vi "Main_12A_X1.vi"() -> ()   [LabVIEW 2024]
uses:
  Utility/Universal Utility/TypeDefs_Utility/Cluster_Row-Column.ctl
  <vilib>/Utility/miscctls.llb/LVMapReplaceAction.ctl
  Utility/Universal Utility/TypeDefs_Utility/ENUM_4 Directions U-D-L-R.ctl
  01caa875-3ad4-4b16-8180-2387dde84b10.vi
  43e758e7-457a-4b0b-abaa-443db623fd74.vi
panel:
  out "Map 2":map{string, map{T1, u32}[]}(c390)
  out "Perimeter 2":map{T1, u32}[](array[numeric])
  out "Area":i32[](array[numeric])
  out "Plant Array":string[](array[string])
  out "Perimeter":u32[](array[numeric])
  out "Map":map{string, T1[]}(c390)
  in  "Example 3":string="RRRRIICCFF\nRRRRIICCCF\nVVRRRCCFFF\nVVRCCCJFFF\nVVVVCJJCFE\nVVIVCCJJEE\nVVIIICJJEE\nMIIIIIJJEE\nMIIISIJEEE\nMMMISSJEEE"
  in  "Example 2":string="OOOOO\nOXOXO\nOOOOO\nOXOXO\nOOOOO"
  in  "Use Puzzle":bool
  out "Answer":u32
  in  "Puzzle":string="WWWWWWWWWWWWWWWWWWHHHHHHHHHHHBYYYYYYYYYYYJJJJJJJJJJJJJJZLLLLLLLLLLLLLLLLLLLLLLBBYBBBBBBBBTTTTKKKKKKKKKKKKKOOOUUUUUUUUUUUSSSSSSSSSSSSSSSSSSSO\nWWWWWWWWWWWWWWWWWWHEHEHHHHHHBBBYYYYYYYYYYJJJJJJJWJJZJZZZZLLLLLLLLLLLLLLLLLLLLLBBBBBBBBBBBBTTTKKKKKKKKKKKKKOOOUUUUUUUUUUUUSSSSSSSSSSSSSSSSSHH\nWWWWWWWWWWWWWWWWWWWEEEHHHHHBBBBBYYYYYYYYYJYJJJJWWJJZZZZZZLLLFFFLLLFLLLHHHHHHHLBBBBBBBBBBBBTTTKKKKKKKKKKKKKOOOOUUUUUUUUUSSSSSSSSSSSSSSSSSSSHH\nWWWWWWWWWWWWWWWWWEEEEEEEEHHBBBSSYYYYYYYYYYYWWWWWWJJZZZZZZLFLFFFFFLFFFLHHHNHHHHABBBBBBBBBBBTTKKKKKKKKKKKKKKOOOUUUUUUUUUUSSSSSSSSSSSSSSSSSHHHH\nWWWWWWWWWWWWWWGEEEEEEEEHEHHHHHHSYYYY..."
  in  "Example 1":string="AAAA\nBBCD\nBBCC\nEEEC"
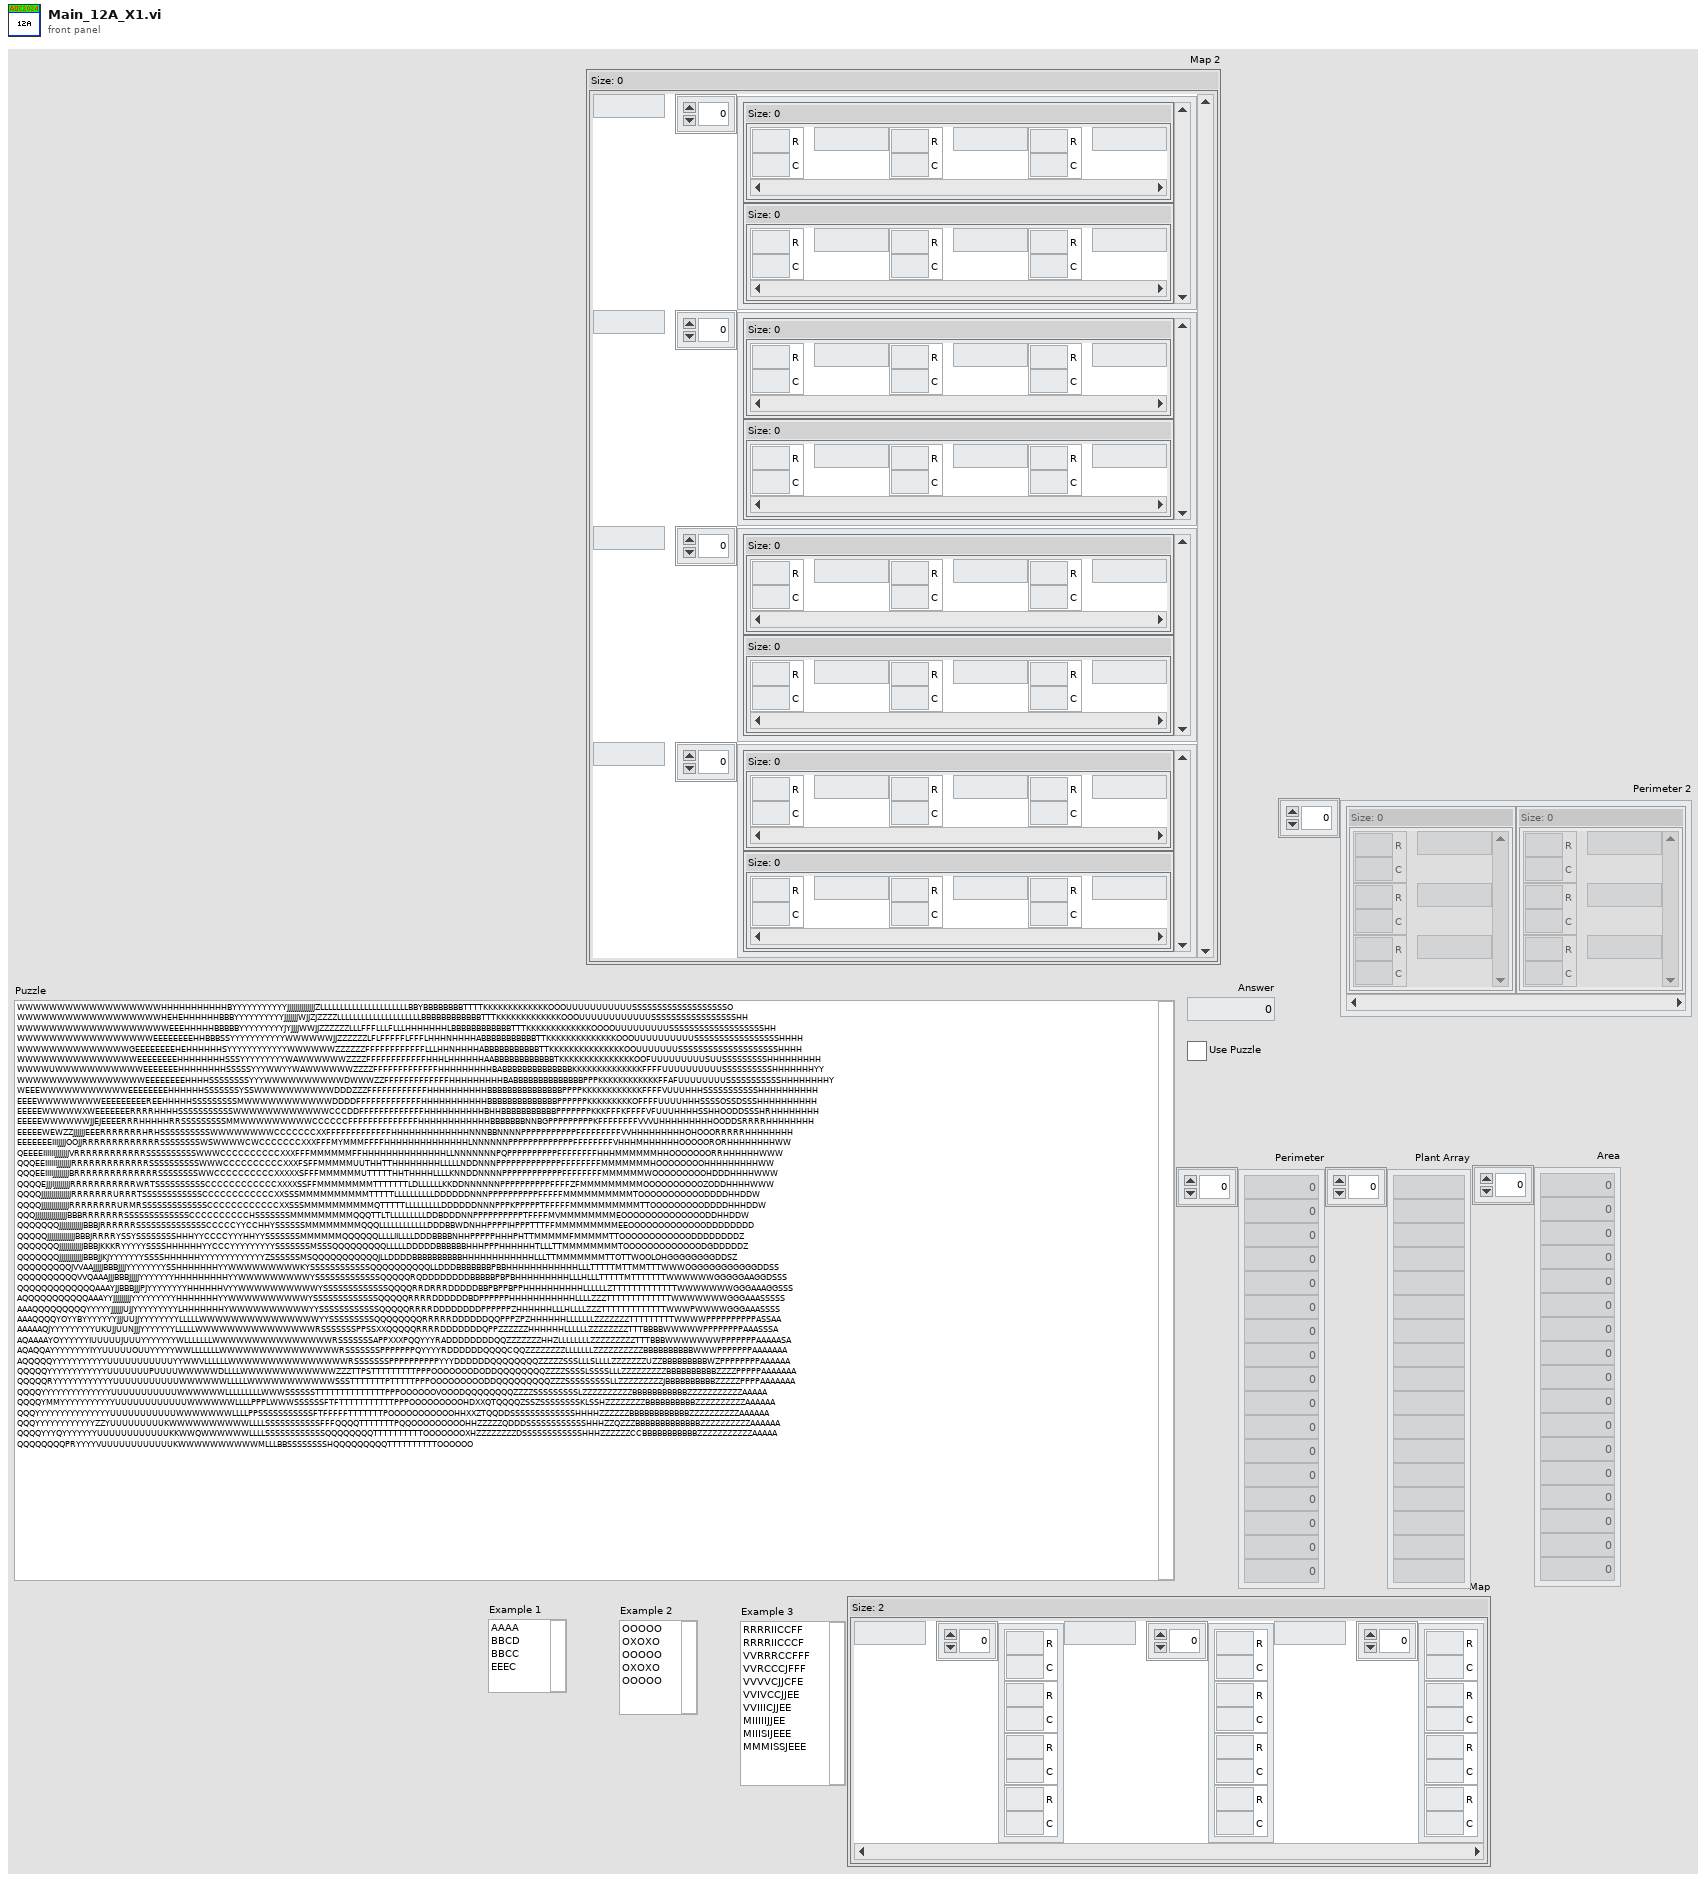
[diagram p1: front panel]
types:
  T1 = typedef "Cluster_Row-Column.ctl" = cluster{"R":i32, "C":i32}
  T2 = typedef "LVMapReplaceAction.ctl" = enum32{"Modify Entry only if found", "Add or Modify Entry", "Delete Entry"}
  T3 = typedef "ENUM_4 Directions U-D-L-R.ctl" = enum16{"Up;-1,0", "Right;0,1", "Down;1,0", "Left;0,-1"}
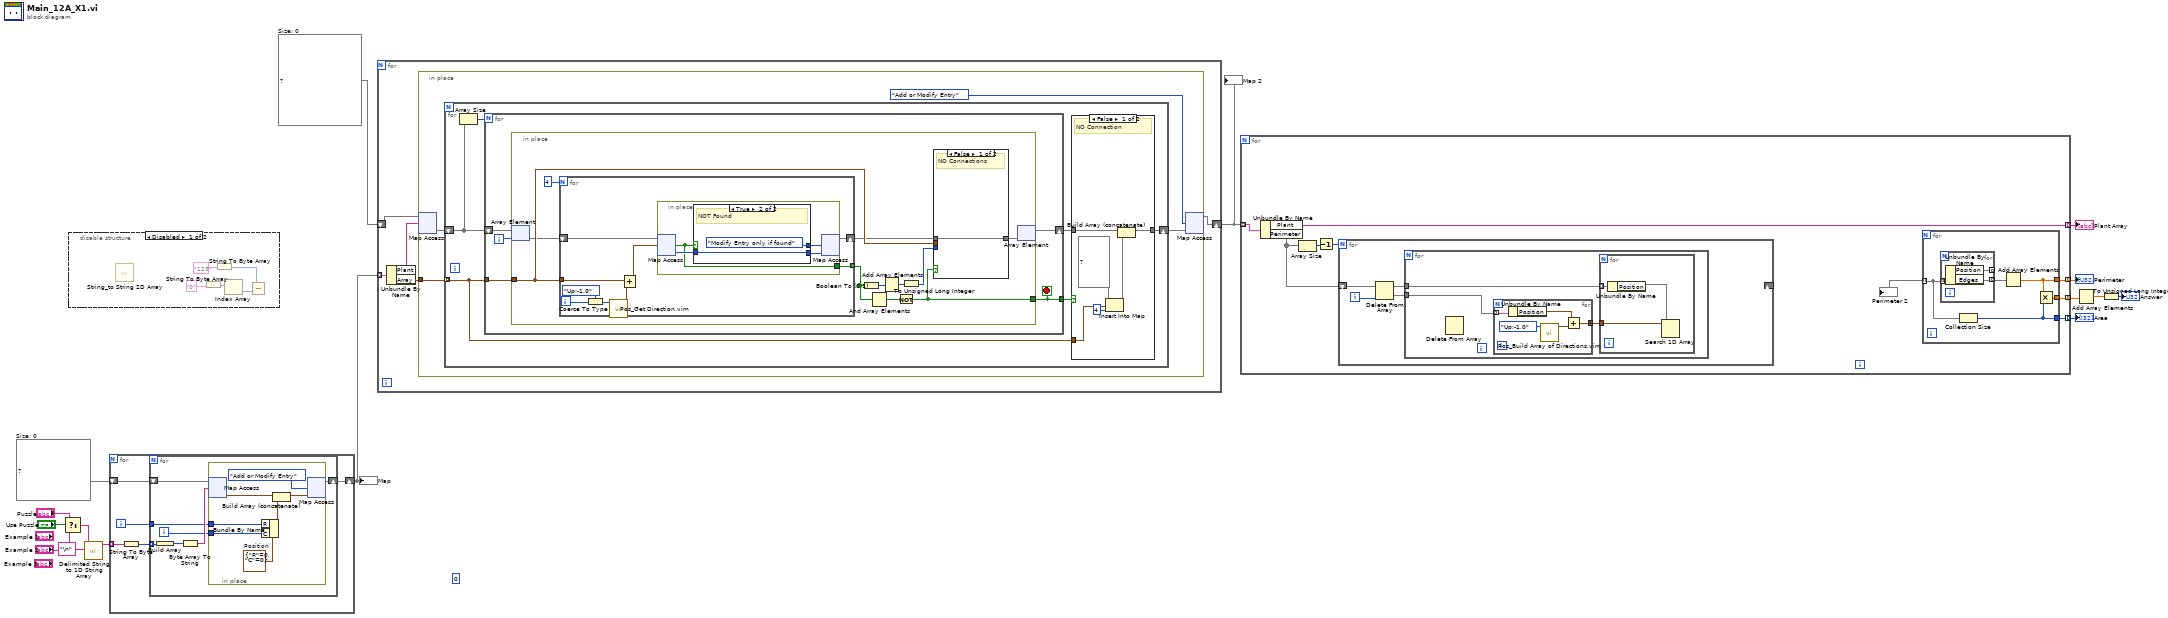
[diagram p0: block diagram]
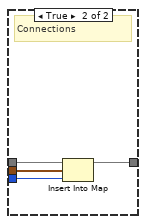
[diagram p3: hidden frame]
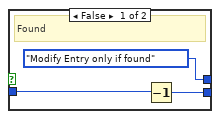
[diagram p4: hidden frame]
diagram:
  w8 = map{string, map{T1, u32}[]} {}  # Size: 0
  w10 = map{string, T1[]} {}  # Size: 0
  (unwired) u32 0 ("number")
  n1 = Select(t="Puzzle", s="Use Puzzle", f="Example 2") -> (s? t:f=w13:string)
  n2 = disable-structure shown="Disabled" {
    frame Disabled {
      n3 = call "String_to String 2D Array.vi"() -> ()  [unwired: 11 in, 1 out]
      n4 = String To Byte Array(string="0") -> (unsigned byte array=w19:u8[])
      n5 = String To Byte Array(string="123") -> (unsigned byte array=w17:u8[])
      n6 = Index Array(array=w19) -> (element=w18:u8)  [unwired: 1 in]
      n7 = Subtract(x=w17, y=w18) -> ()  [unwired: 1 out]
    }
    frame Enabled {
    }
  }
  n8 = call <vilib>:"Delimited String to 1D String Array.vi"("delimiter"="\n" ("delimiter (Tab)"), "delimited string"=w13) -> ("string array"=w15:string[])  [unwired: 9 in]
  n9 = for {
    tunnel: w15 -> [w26] mode=indexing
    shift-right: [w23] -> w9
    shift-left: w10 -> [w24]
    i -> [w22]
    n10 = String To Byte Array(string=w26) -> (unsigned byte array=w25:u8[])
    n11 = for {
      tunnel: w25 -> [w33] mode=indexing
      shift-right: [w30] -> w23
      shift-left: w24 -> [w31]
      tunnel: w22 -> [w28]
      i -> [w27]
      n12 = Build Array(w33) -> (w32:u8[])
      n13 = Byte Array To String(unsigned byte array=w32) -> (string=w29:string)
      n14 = in-place {
        in-place-border: w28 -> [w38]
        in-place-border: w27 -> [w37]
        w39 = T1 {"R"=0, "C"=0}  # Position
        n15 = in-place-map #1(w31, w29) -> (w36:T1[])  [unwired: 1 in, 1 out]
        n16 = Bundle By Name(cluster=w39, "R"=w38, "C"=w37) -> (w34:T1)
        n17 = Build Array (concatenate)(w36, w34) -> (w35:T1[])
        n18 = in-place-map #1(w35, LVMapReplaceAction."Add or Modify Entry" ("action")) -> (w30:map{string, T1[]})  [unwired: 2 out]
      }
    }
  }
  "Map" <- w9
  n19 = for {
    tunnel: w9 -> [w45] mode=indexing
    shift-right: [w43] -> w7
    shift-left: w8 -> [w44]
    n20 = Unbundle By Name(w45) -> ("Plant"=w42:string, "Array"=w41:T1[])
    n21 = in-place {
      in-place-border: w41 -> [w48]
      n22 = in-place-map #2(w44, w42) -> (w47:map{T1, u32}[])  [unwired: 1 in, 1 out]
      n23 = for {
        tunnel: w48 -> [w50] mode=indexing
        shift-right: [w51] -> w46
        shift-left: w47 -> [w55]
        n24 = Array Size(array=w55) -> (size(s)=w54:i32)
        n25 = for {
          N: w54 -> [_]
          tunnel: w50 -> [w67]
          shift-right: [w64] -> w52
          shift-left: w55 -> [w66]
          tunnel: [w63] -> w53
          i -> [w65]
          stop <- w63 stop-if-true
          n26 = in-place {
            in-place-border: w67 -> [w78]
            in-place-border: [w68] -> w63
            n27 = in-place-array #3(w66, w65) -> (w73:map{T1, u32})
            n28 = for {
              N: 4 -> [_]
              tunnel: w78 -> [w86]
              shift-right: [w85] -> w76
              shift-left: w73 -> [w88]
              tunnel: [w84] -> w71 mode=indexing
              i -> [w90]
              n29 = Coerce To Type(0:w90, 1:ENUM_4_Directions_U-D-L-R."Up;-1,0" ("Direction")) -> (2:w92:T3)
              n30 = call "Pos_Get Direction.vim"("Direction 2"=w92) -> ("Direction"=w89:T1)  [unwired: 10 in]
              n31 = Add(x=w86, y=w89) -> (x+y=w87:T1)
              n32 = in-place {
                in-place-border: [w95] -> w84
                n33 = in-place-map #4(w88, w87) -> (w96:u32, w95:bool)  [unwired: 1 in]
                n34 = case shown="True" w95 {
                  tunnel: w96 -> [w99 w101]
                  tunnel: [w98 w101] -> w94
                  tunnel: [LVMapReplaceAction."Modify Entry only if found" ("action") LVMapReplaceAction."Modify Entry only if found" ("action")] -> w93
                  frame False {
                    # "Found"
                    n35 = Decrement(x=w99) -> (x-1=w98:u32)
                  }
                  frame True {
                    # "NOT Found"
                  }
                }
                n36 = in-place-map #4(w94, w93) -> (w85:map{T1, u32})  [unwired: 2 out]
              }
            }
            n37 = Boolean To (0,1)(Boolean=w71) -> (0, 1=w75:i16[])
            n38 = And Array Elements(Boolean array=w71) -> (logical AND=w69:bool)
            n39 = Add Array Elements(numeric array=w75) -> (sum=w74:i16)
            n40 = Not(x=w69) -> (.not. x?=w68:bool)
            n41 = To Unsigned Long Integer(number=w74) -> (unsigned 32bit integer=w70:u32)
            n42 = case shown="False" w68 {
              tunnel: w78 -> [_ w83]
              tunnel: w76 -> [w79 w82]
              tunnel: [w79 w81] -> w72
              tunnel: w70 -> [_ w80]
              frame False {
                # "NO Connections"
              }
              frame True {
                # "Connections"
                n43 = Insert Into Map(map in=w82, key=w83, value=w80) -> (map out=w81:map{T1, u32})  [unwired: 2 out]
              }
            }
            n44 = in-place-array #3(w72) -> (w64:map{T1, u32}[])  [unwired: 1 out]
          }
        }
        n45 = case shown="False" w53 {
          tunnel: w52 -> [w61 w62]
          tunnel: [w60 w62] -> w51
          tunnel: w50 -> [w57 _]
          frame False {
            # "NO Connection"
            n46 = Insert Into Map(map in=map{T1, u32} {} ("Perimeter"), key=w57, value=u32 4) -> (map out=w58:map{T1, u32})  [unwired: 2 out]
            n47 = Build Array (concatenate)(w61, w58) -> (w60:map{T1, u32}[])
          }
          frame True {
            # "Connection"
          }
        }
      }
      n48 = in-place-map #2(w46, LVMapReplaceAction."Add or Modify Entry" ("action")) -> (w43:map{string, map{T1, u32}[]})  [unwired: 2 out]
    }
  }
  "Map 2" <- w7
  n49 = for {
    tunnel: w7 -> [w110] mode=indexing
    tunnel: [w109] -> w3 mode=indexing
    tunnel: [w108] -> w4 mode=indexing
    tunnel: [w107] -> w2 mode=indexing
    tunnel: [w106] -> w6 mode=indexing
    n50 = Unbundle By Name(w110) -> ("Plant"=w109:string, "Perimeter"=w104:map{T1, u32}[])
    n51 = Array Size(array=w104) -> (size(s)=w103:i32)
    n52 = Decrement(x=w103) -> (x-1=w102:i32)
    n53 = for {
      N: w102 -> [_]
      shift-right: _ -> [_]
      shift-left: w104 -> [w114]
      i -> [w111]
      n54 = Delete From Array(array=w114, index=w111) -> (deleted portion=w113:map{T1, u32}, array with subset deleted=w112:map{T1, u32}[])  [unwired: 1 in]
      n55 = for {
        tunnel: w113 -> [w117]
        tunnel: w112 -> [w116]
        n56 = Delete From Array() -> ()  [unwired: 3 in, 2 out]
        n57 = for {
          tunnel: w117 -> [w125] mode=indexing
          tunnel: [w121] -> w115 mode=concatenating
          n58 = Unbundle By Name(w125) -> ("Position"=w122:T1)
          n59 = call "Pos_Build Array of Directions.vim"("Direction"=ENUM_4_Directions_U-D-L-R."Up;-1,0") -> ("Direction Positions Out"=w123:T1[])  [unwired: 10 in]
          n60 = Add(x=w122, y=w123) -> (x+y=w121:T1[])
        }
        n61 = for {
          tunnel: w116 -> [w120] mode=indexing
          tunnel: w115 -> [w119]
          n62 = Unbundle By Name(w120) -> ("Position"=w118)
          n63 = Search 1D Array(1D array=w119, element=w118) -> ()  [unwired: 1 in, 1 out]
        }
      }
    }
    n64 = for {
      tunnel: [w129] -> w108
      tunnel: [w128] -> w107
      tunnel: [w127] -> w106
      tunnel: [w126] -> w105 mode=indexing
      n65 = for {
        tunnel: w126 -> [w133] mode=indexing
        tunnel: [w132] -> w130 mode=indexing
        tunnel: [w131] -> _ mode=indexing
        n66 = Unbundle By Name(w133) -> ("Position"=w131, "Edges"=w132)
      }
      n67 = Collection Size(1:w126) -> (0:w128:i32)
      n68 = Add Array Elements(numeric array=w130) -> (sum=w129:dbl)
      n69 = Multiply(x=w129, y=w128) -> (x*y=w127:dbl)
    }
    "Perimeter 2" <- w105
  }
  "Perimeter" <- w4
  "Plant Array" <- w3
  "Area" <- w2
  n70 = Add Array Elements(numeric array=w6) -> (sum=w5:dbl)
  n71 = To Unsigned Long Integer(number=w5) -> (unsigned 32bit integer=→"Answer":u32)
